vi "SerializeTree.vi"(8 "error in (no error)":errorcluster, 9 "TagToPathMap":T1[](array[typedef]), 10 "Tag":string, 11 "Tree Refnum":refnum<vi>) -> (0 "error out":errorcluster, 3 "Formatted JSON string":string)   [LabVIEW 2017, in "TreeSerializer.lvlib"]
uses:
  TreeSerializer.lvlib
  KeyValuePair.ctl
  Constants.vi
  JsonFormatter/JsonFormatter.lvlib
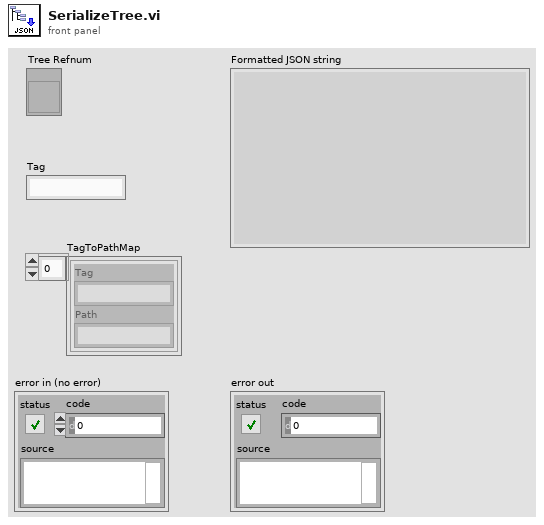
[diagram p1: front panel]
types:
  T1 = typedef "TreeSerializer.lvlib/KeyValuePair.ctl" = cluster{"Tag":string, "Path":string}
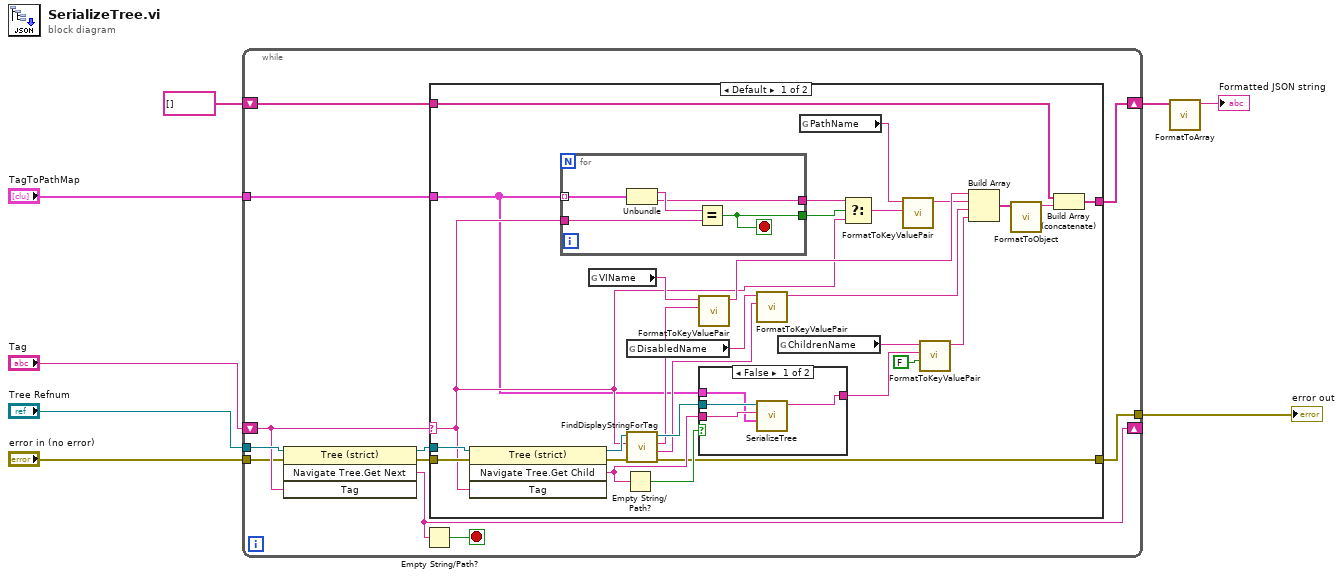
[diagram p0: block diagram]
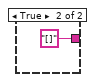
[diagram p2: hidden frame]
diagram:
  n1 = while {
    tunnel: "Tree Refnum" -> [w17]
    shift-right: [w18] -> _
    shift-left: "Tag" -> [w13]
    shift-right: [w15] -> w6
    shift-left: string[] [] -> [w16]
    tunnel: "TagToPathMap" -> [w12]
    tunnel: "error in (no error)" -> [w11]
    tunnel: [w9] -> w1
    stop <- w19 stop-if-true
    n2 = invoke class="Tree (strict)" method="Navigate Tree.Get Next"(reference=w17, error in=w11, "Tag"=w13) -> (reference out=w14:refnum<vi>, error out=w10:errorcluster, "Navigate Tree:Get Next Item"=w18:string)  [unwired: 1 in, 1 out]
    n3 = Empty String/Path?(string/path=w18) -> (empty?=w19:bool)
    n4 = case shown="Default" w13 {
      selector: w13 -> [w22 _]
      tunnel: w14 -> [w46 _]
      tunnel: w16 -> [w44 w60]
      tunnel: [w43 w60] -> w15
      tunnel: w12 -> [w20 _]
      tunnel: w10 -> [w27 w59]
      tunnel: [w25 w59] -> w9
      frame Default {
        n5 = invoke class="Tree (strict)" method="Navigate Tree.Get Child"(reference=w46, error in=w27, "Tag"=w22) -> (reference out=w45:refnum<vi>, error out=w26:errorcluster, "Navigate Tree:Get Child"=w48:string)  [unwired: 1 in, 1 out]
        n6 = for {
          tunnel: w20 -> [w53] mode=indexing
          tunnel: w22 -> [w51]
          tunnel: [w49] -> w23
          tunnel: [w50] -> w24
          stop <- w50 stop-if-true
          n7 = Unbundle(w53) -> ("Tag"=w52:string, "Path"=w49:string)
          n8 = Equal?(x=w52, y=w51) -> (x = y?=w50:bool)
        }
        n9 = global read "Constants.vi" "VIName"() -> (w41:string)
        n10 = Empty String/Path?(string/path=w48) -> (empty?=w47:bool)
        n11 = global read "Constants.vi" "DisabledName"() -> (w30:string)
        n12 = call "FindDisplayStringForTag.vi"("error in (no error)"=w26, "Tag"=w22, "Tree Refnum"=w45) -> ("error out"=w25:errorcluster, "Disabled"=w28:string, "Display String"=w40:string, "Tree Refnum out"=w42:refnum<vi>)  [unwired: 5 in]
        n13 = call "FormatToKeyValuePair.vi"("Value"=w40, "Key"=w41) -> ("Formatted string"=w39:string)  [unwired: 9 in]
        n14 = case shown="False" w47 {
          tunnel: w42 -> [w57 _]
          tunnel: w48 -> [w56 _]
          tunnel: [w55 "[]" ("JSON object")] -> w35
          tunnel: w20 -> [w54 _]
          frame False {
            n15 = call "SerializeTree.vi"("TagToPathMap"=w54, "Tag"=w56, "Tree Refnum"=w57) -> ("Formatted JSON string"=w55:string)  [unwired: 7 in, 1 out]
          }
          frame True {
          }
        }
        n16 = call "FormatToKeyValuePair.vi"("Value"=w28, "Key"=w30) -> ("Formatted string"=w29:string)  [unwired: 9 in]
        n17 = global read "Constants.vi" "ChildrenName"() -> (w36:string)
        n18 = global read "Constants.vi" "PathName"() -> (w38:string)
        n19 = Select(t=w23, s=w24, f=w22) -> (s? t:f=w21:string)
        n20 = call "FormatToKeyValuePair.vi"("Value"=w21, "Key"=w38) -> ("Formatted string"=w37:string)  [unwired: 9 in]
        n21 = call "FormatToKeyValuePair.vi"("Escape Value string?"=FALSE ("Escape Value?"), "Value"=w35, "Key"=w36) -> ("Formatted string"=w33:string)  [unwired: 8 in]
        n22 = Build Array(w39, w37, w29, w33) -> (w32:string[])
        n23 = call "FormatToObject.vi"("Properties"=w32) -> ("Formatted string"=w31:string)  [unwired: 10 in]
        n24 = Build Array (concatenate)(w44, w31) -> (w43:string[])
      }
      frame "" {
      }
    }
  }
  "error out" <- w1
  n25 = call "FormatToArray.vi"("Array"=w6) -> ("Formatted string"=→"Formatted JSON string":string)  [unwired: 10 in]
